vi "ReadFilesOnMP.vi"(11 "VISA":refnum<visa-resource-name>) -> ()   [LabVIEW 2016]
uses:
  ColorText/Code.xctl
panel:
  in  "File Listing":i32(listbox)
  out "Code":string(xcontrol)
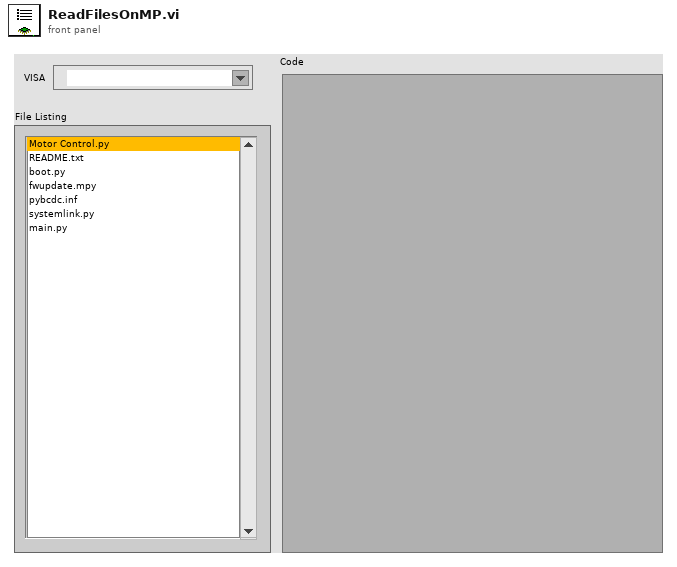
[diagram p1: front panel]
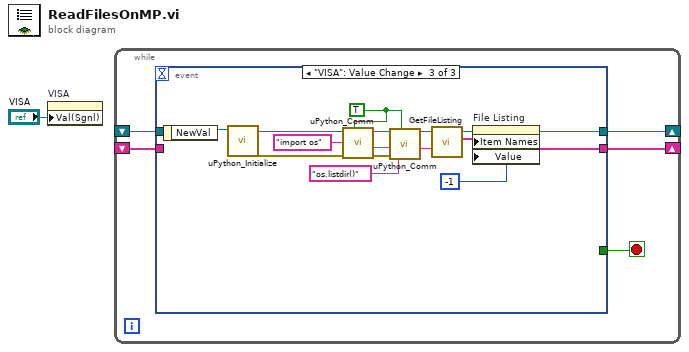
[diagram p0: block diagram]
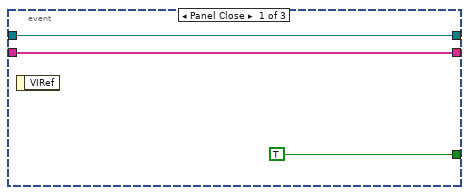
[diagram p2: hidden frame]
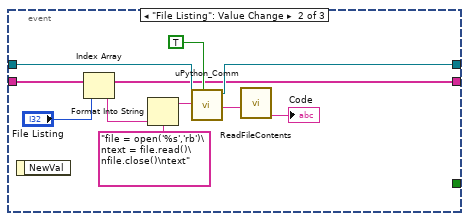
[diagram p3: hidden frame]
diagram:
  n1 = property on="VISA" class="VISAName"("Val(Sgnl)"="VISA") -> ()  [unwired: 2 in, 2 out]
  n2 = while {
    shift-right: [w3] -> _
    shift-left: _ -> [w4]
    shift-right: [w2] -> _
    shift-left: _ -> [w5]
    stop <- w6 stop-if-true
    n3 = event shown="[2] \"VISA\": Value Change" {
      selector: _ -> [_ _ _]
      dyn-events: _ -> [_ _ _]
      timeout: _ -> [_ _ _]
      tunnel: [TRUE _ _] -> w6
      tunnel: w5 -> [w7 w10 _]
      tunnel: w4 -> [w8 w18 _]
      tunnel: [w8 w11 w22] -> w3
      tunnel: [w7 w10 w21] -> w2
      event Panel Close {
        n4 = event-data() -> ()  [unwired: 1 in, 1 out]
      }
      event "File Listing": Value Change {
        n5 = event-data() -> ()  [unwired: 1 in, 1 out]
        n6 = Index Array(array=w10, index="File Listing") -> (element=w13:string)
        n7 = Format Into String(format string="file = open('%s','rb')\ntext = file.read()\nfile.close()\ntext" ("write buffer"), w13) -> (resulting string=w12:string)  [unwired: 2 in, 1 out]
        n8 = call "uPython_Comm.vi"("Wait for Reply?"=TRUE, "Script"=w12, "VISA Refnum in"=w18) -> ("Console Out"=w16:string, "VISA out"=w11:refnum<visa-resource-name>)  [unwired: 4 in, 3 out]
        n9 = call "ReadFileContents.vi"("Console"=w16) -> ("File Contents"=→"Code":string)  [unwired: 9 in, 1 out]
      }
      event "VISA": Value Change {
        w25 = TRUE ("Wait for Reply?")
        n10 = event-data() -> ("NewVal"=w20:refnum<visa-resource-name>)  [unwired: 1 in]
        n11 = call "uPython_Initialize.vi"("VISA Refnum in"=w20) -> ("error out"=w32:errorcluster, "VISA Refnum out"=w31:refnum<visa-resource-name>)  [unwired: 9 in]
        n12 = call "uPython_Comm.vi"("Wait for Reply?"=w25, "error in (no error)"=w32, "Script"="import os" ("element"), "VISA Refnum in"=w31) -> ("error out"=w27:errorcluster, "Console Out"=w28:string, "VISA out"=w29:refnum<visa-resource-name>)  [unwired: 3 in, 2 out]
        n13 = call "uPython_Comm.vi"("Wait for Reply?"=w25, "error in (no error)"=w27, "Console In"=w28, "Script"="os.listdir()" ("element"), "VISA Refnum in"=w29) -> ("Console Out"=w30:string, "VISA out"=w22:refnum<visa-resource-name>)  [unwired: 2 in, 3 out]
        n14 = call "GetFileListing.vi"("Console In"=w30) -> ("Files"=w21:string[])  [unwired: 9 in, 1 out]
        n15 = property on="File Listing" class="LstBox (strict)"("Item Names"=w21, "Value"=-1 ("File Listing")) -> ()  [unwired: 2 in, 2 out]
      }
    }
  }
